vi "set_pixel_dwell_time.vi"(8 "error in (no error)":errorcluster, 10 "Pixel dwell time":dbl, 11 "FPGAWrapperRK110512Fiber_Spiral in":refnum<class "FPGAWrapperRK110512Fiber_Spiral.lvclass">) -> (0 "error out":errorcluster, 3 "FPGAWrapperRK110512Fiber_Spiral out":refnum<class "FPGAWrapperRK110512Fiber_Spiral.lvclass">)   [LabVIEW 2010, in "FPGAWrapperRK110512Fiber_Spiral.lvclass"]
uses:
  FPGAWrapperRK110512Fiber_Spiral.lvclass
  FPGAWrapperRK110512Fiber_Spiral.lvclass/FPGAWrapperRK110512Fiber_Spiral.ctl
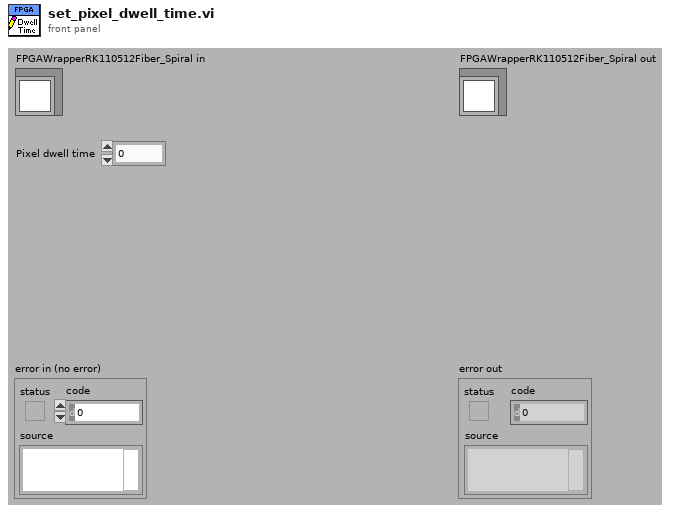
[diagram p1: front panel]
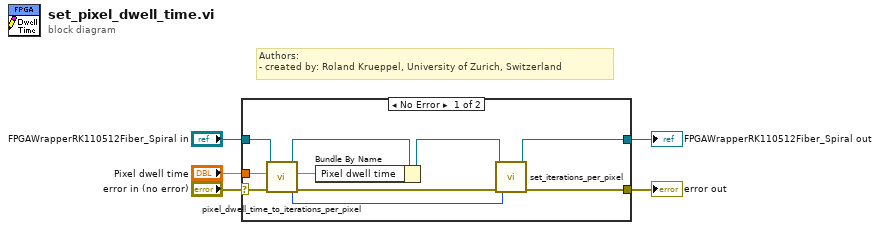
[diagram p0: block diagram]
diagram:
  # "Authors: \n- created by: Roland Krueppel, University of Zurich, Switzerland"
  n1 = case shown="No Error" "error in (no error)" {
    selector: "error in (no error)" -> [w13 w16]
    tunnel: [w9 w16] -> w4
    tunnel: [w7 w17] -> w2
    tunnel: "FPGAWrapperRK110512Fiber_Spiral in" -> [w15 w17]
    tunnel: "Pixel dwell time" -> [w12 _]
    frame No Error {
      n2 = call-dynamic "pixel_dwell_time_to_iterations_per_pixel.vi"("error in (no error)"=w13, "Pixel dwell time"=w12, "FPGAWrapperRK110512Fiber_Spiral in"=w15) -> ("error out"=w10:errorcluster, "Iterations per pixel"=w6:i32, "Pixel dwell time"=w11:dbl, "FPGAWrapperRK110512Fiber_Spiral out"=w14:refnum<class "FPGAWrapperRK110512Fiber_Spiral.lvclass">)  [unwired: 5 in]
      n3 = Bundle By Name(cluster=w14, "Pixel dwell time"=w11) -> (w8:refnum<class "FPGAWrapperRK110512Fiber_Spiral.lvclass">)
      n4 = call-dynamic "set_iterations_per_pixel.vi"("error in (no error)"=w10, "iterations per pixel"=w6, "FPGAWrapperRK120511Fiber_Spiral in"=w8) -> ("error out"=w9:errorcluster, "FPGAWrapperRK120511Fiber_Spiral out"=w7:refnum<class "FPGAWrapperRK110512Fiber_Spiral.lvclass">)  [unwired: 7 in]
    }
    frame Error {
    }
  }
  "error out" <- w4
  "FPGAWrapperRK110512Fiber_Spiral out" <- w2
